vi "Initialize DIDPID Cluster.vi"(8 "error in":errorcluster, 9 "Lookup":variant, 10 "DIDs/PIDs":T1[](array[typedef]) {"Signals"."Byte Order" items=["Little Endian", "Big Endian"]; "Signals"."Data Type" items=["Signed", "Unsigned", "IEEE Float"]}, 11 "Cluster In":refnum<k21>) -> (0 "error out":errorcluster, 1 "Lookup":variant, 3 "Cluster Out":refnum<k21>)   [LabVIEW 2015, in "Diagnostics Addon Engine.lvlib"]
uses:
  Diagnostics Addon Engine.lvlib
  Shared/Types/Common Frame Parameters.ctl
  Shared/Types/MessageType Selector.ctl
  Shared/Types/Signal Parameters.ctl
  Shared/Types/CAN Frame.ctl
  <vilib>/xnet/xnet.llb/XNET Create Session (Conversion).vi
  Shared/SubVIs/GUID Lookup.vi
  Shared/Diagnostics Addon Shared.lvlib
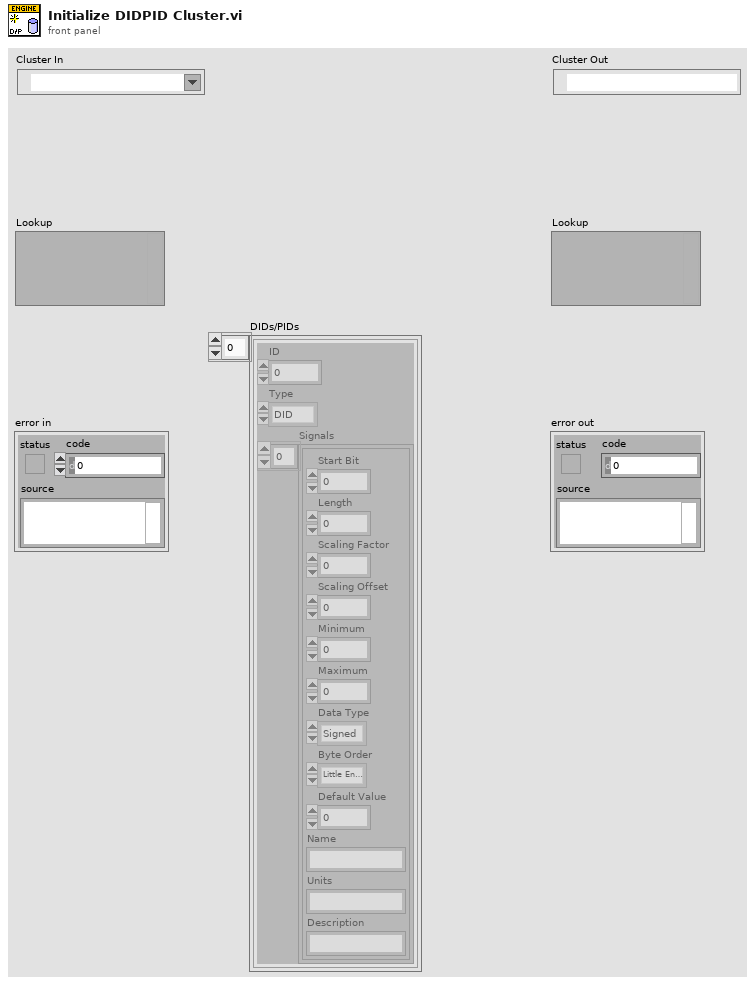
[diagram p1: front panel]
types:
  T1 = typedef "Diagnostics Addon Shared.lvlib/Common Frame Parameters.ctl" = cluster{"ID":u32, "Type":T2, "Signals":T3[]}
  T2 = typedef "Diagnostics Addon Shared.lvlib/MessageType Selector.ctl" = enum16{"DID", "CDID", "PID", "CPID", "Read Memory", "Write Memory", "DTC Control", "IO Cmd", "IO Resp", "Routine Start Cmd", "Routine Start Resp", "Routine Request Cmd", "Routine Request Resp", "Routine Stop Cmd", "Routine Stop Resp"}
  T3 = typedef "Diagnostics Addon Shared.lvlib/Signal Parameters.ctl" = cluster{"Start Bit":u8, "Length":u8, "Scaling Factor":dbl, "Scaling Offset":dbl, "Minimum":dbl, "Maximum":dbl, "Data Type":u32, "Byte Order":u32, "Default Value":dbl, "Name":string, "Units":string, "Description":string}
  T4 = typedef "Diagnostics Addon Shared.lvlib/CAN Frame.ctl" = cluster{"Frame name":string, "Identifier":u32, "Payload Length":u32, "Timing Type":u32, "Transmit Time":dbl, "Extended Identifier?":bool, "Comment":string}
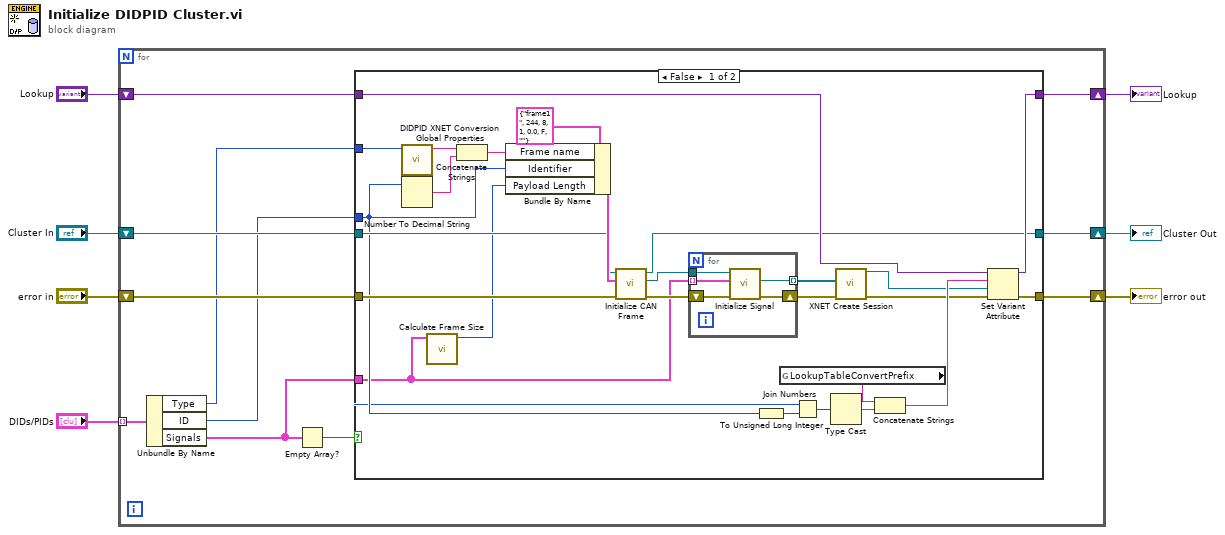
[diagram p0: block diagram]
diagram:
  n1 = for {
    shift-right: [w17] -> w6
    shift-left: "error in" -> [w14]
    tunnel: "DIDs/PIDs" -> [w18] mode=indexing
    shift-right: [w15] -> w4
    shift-left: "Lookup" -> [w16]
    shift-right: [w12] -> w1
    shift-left: "Cluster In" -> [w13]
    n2 = Unbundle By Name(w18) -> ("Type"=w10:T2, "ID"=w11:u32, "Signals"=w9:T3[])
    n3 = Empty Array?(array=w9) -> (empty?=w8:bool)
    n4 = case shown="False" w8 {
      tunnel: [w44 w52] -> w17
      tunnel: w16 -> [w43 w50]
      tunnel: [w42 w50] -> w15
      tunnel: w14 -> [w40 w52]
      tunnel: w13 -> [w34 w51]
      tunnel: [w32 w51] -> w12
      tunnel: w11 -> [w30 _]
      tunnel: w10 -> [w29 _]
      tunnel: w9 -> [w20 _]
      frame False {
        n5 = call "DIDPID XNET Conversion Global Properties.vi"("DID/PID Selector"=w29) -> ("signal name"=w38:string)  [unwired: 9 in, 1 out]
        n6 = Number To Decimal String(number=w30) -> (decimal integer string=w31:string)  [unwired: 1 in]
        n7 = call "Calculate Frame Size.vi"("Parameters"=w20) -> ("Bytes"=w19:u16)  [unwired: 10 in]
        n8 = Concatenate Strings(w38, w31) -> (w37:string)
        n9 = Bundle By Name(cluster=T4 {"Frame name"="frame1", "Identifier"=244, "Payload Length"=8, "Timing Type"=1, "Transmit Time"=0.0, "Extended Identifier?"=FALSE, "Comment"=""} ("CAN Frame"), "Frame name"=w37, "Identifier"=w30, "Payload Length"=w19) -> (w35:T4)
        n10 = call "Initialize CAN Frame.vi"("error in"=w40, "CAN Frame"=w35, "cluster in"=w34) -> ("error out"=w39:errorcluster, "frame out"=w33:refnum<k21>, "cluster out"=w32:refnum<k21>)  [unwired: 6 in]
        n11 = for {
          tunnel: w33 -> [w45]
          tunnel: w20 -> [w46] mode=indexing
          shift-right: [w48] -> w41
          shift-left: w39 -> [w49]
          tunnel: [w47] -> w28 mode=indexing
          n12 = call "Initialize Signal.vi"("error in"=w49, "Signal"=w46, "frame in"=w45) -> ("error out"=w48:errorcluster, "signal out"=w47:refnum<k21>)  [unwired: 6 in, 1 out]
        }
        n13 = To Unsigned Long Integer(number=w30) -> (unsigned 32bit integer=w22:u32)
        n14 = global read "GUID Lookup.vi" "LookupTableConvertPrefix"() -> (w27:string)
        n15 = Join Numbers(hi=w29, lo=w22) -> ((hi.lo)=w21:u64)
        n16 = Type Cast(x=w21) -> (*(type *) &x=w23:string)  [unwired: 1 in]
        n17 = call-poly <vilib>:"XNET Create Session.vi"("signal list"=w28, "error in (no error)"=w41) -> ("session out"=w24:refnum<k21>, "error out"=w25:errorcluster)  [unwired: 1 in, 11 out]
        n18 = Concatenate Strings(w27, w23) -> (w26:string)
        n19 = Set Variant Attribute(Variant=w43, name=w26, value=w24, error in=w25) -> (Variant out=w42:variant, error out=w44:errorcluster)  [unwired: 1 out]
      }
      frame True {
      }
    }
  }
  "error out" <- w6
  "Cluster Out" <- w1
  "Lookup" <- w4
